vi "Resize Pane.vi"(6 "Pane size":i32, 8 "error in (no error)":errorcluster, 11 "IObject in":refnum<class "IObject.lvclass">) -> (0 "error out":errorcluster, 2 "Resized?":bool, 3 "IObject out":refnum<class "IObject.lvclass">)   [LabVIEW 2021, in "IObject.lvclass"]
uses:
  IObject.lvclass
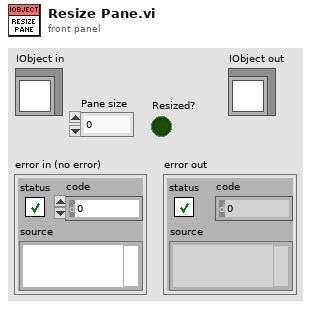
[diagram p1: front panel]
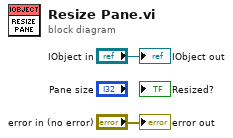
[diagram p0: block diagram]
diagram:
  "error out" <- "error in (no error)"
  "IObject out" <- "IObject in"
